vi "CopyToZip.vi"(4 "FTP Client":u16(ring) items=["VMMC", "U_HI", "Sloan Kett", "Columbia", "RRI Test"], 7 "directory path":path=path "D:/") -> ()   [LabVIEW 2022 SP3]
uses:
  <vilib>/Utility/SMTP/NI_SMTPEmail.lvlib
panel:
  out "spreadsheet string":string
  # "Save to Zip in progress. Report errors to RRI."
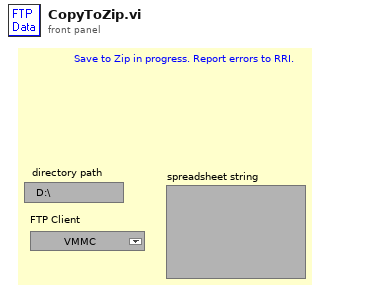
[diagram p1: front panel]
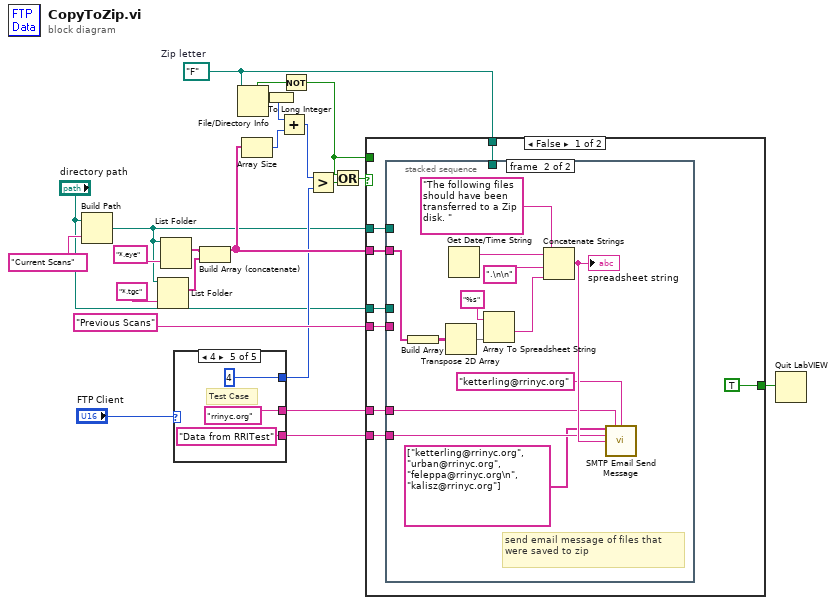
[diagram p0: block diagram]
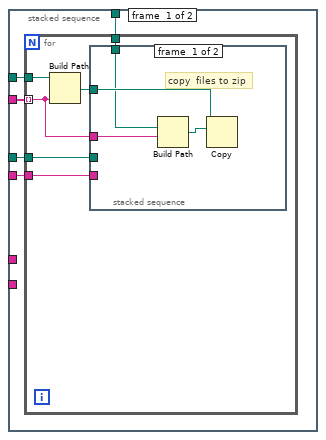
[diagram p2: hidden frame]
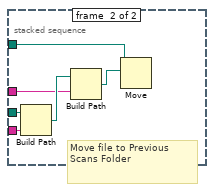
[diagram p3: hidden frame]
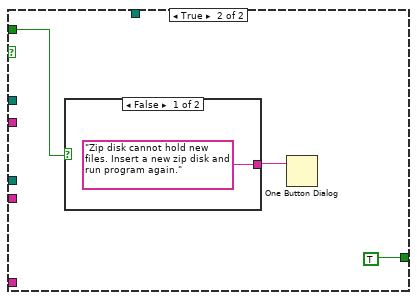
[diagram p4: hidden frame]
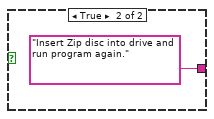
[diagram p5: hidden frame]
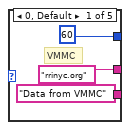
[diagram p6: hidden frame]
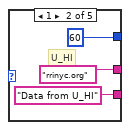
[diagram p7: hidden frame]
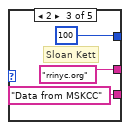
[diagram p8: hidden frame]
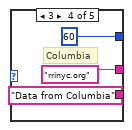
[diagram p9: hidden frame]
diagram:
  w15 = path "F:/"  # Zip letter
  n1 = Build Path(base path="directory path", name or relative path="Current Scans") -> (appended path=w9:path)
  n2 = List Folder(path=w9, pattern="*.tgc") -> (filenames=w18:string[])  [unwired: 1 in, 4 out]
  n3 = List Folder(path=w9, pattern="*.eye") -> (filenames=w19:string[])  [unwired: 1 in, 4 out]
  n4 = case shown="4" "FTP Client" {
    tunnel: ["Data from VMMC" "Data from U_HI" "Data from MSKCC" "Data from Columbia" "Data from RRITest"] -> w17
    tunnel: ["rrinyc.org" "rrinyc.org" "rrinyc.org" "rrinyc.org" "rrinyc.org"] -> w16
    tunnel: [60 60 100 60 4] -> w10
    frame 0, Default {
      # "VMMC"
    }
    frame 1 {
      # "U_HI"
    }
    frame 2 {
      # "Sloan Kett"
    }
    frame 3 {
      # "Columbia"
    }
    frame 4 {
      # "Test Case"
    }
  }
  n5 = Build Array (concatenate)(w19, w18) -> (w14:string[])
  n6 = File/Directory Info(path=w15) -> (directory=w5:bool, size=w1:i64)  [unwired: 1 in, 5 out]
  n7 = Array Size(array=w14) -> (size(s)=w12:i32)
  n8 = To Long Integer(number=w1) -> (32bit integer=w13:i32)
  n9 = Add(x=w13, y=w12) -> (x+y=w11:i32)
  n10 = Not(x=w5) -> (.not. x?=w2:bool)
  n11 = Greater?(x=w11, y=w10) -> (0:w3:bool)
  n12 = Or(x=w2, y=w3) -> (x .or. y?=w4:bool)
  n13 = case shown="False" w4 {
    tunnel: w9 -> [w46 _]
    tunnel: "Previous Scans" -> [w45 _]
    tunnel: w17 -> [w44 _]
    tunnel: w16 -> [w43 _]
    tunnel: w15 -> [w42 _]
    tunnel: w14 -> [w41 _]
    tunnel: [TRUE TRUE] -> w7
    tunnel: "directory path" -> [w39 _]
    tunnel: w2 -> [_ w81]
    frame False {
      n14 = stacked-sequence {
        tunnel: w45 -> [w51 _]
        tunnel: w46 -> [w50 _]
        tunnel: w41 -> [w49 w80]
        tunnel: w44 -> [_ w70]
        tunnel: w43 -> [_ w69]
        tunnel: w42 -> [w48 _]
        tunnel: w39 -> [w47 _]
        frame #0 {
          n15 = for {
            tunnel: w49 -> [w55] mode=indexing
            tunnel: w50 -> [w53]
            tunnel: w51 -> [w56]
            tunnel: w48 -> [w54]
            tunnel: w47 -> [w52]
            n16 = Build Path(base path=w53, name or relative path=w55) -> (appended path=w57:path)
            n17 = stacked-sequence {
              tunnel: w57 -> [w61 w62]
              tunnel: w52 -> [_ w67]
              tunnel: w56 -> [_ w66]
              tunnel: w55 -> [w60 w63]
              tunnel: w54 -> [w58 _]
              frame #0 {
                # "copy  files to zip"
                n18 = Build Path(base path=w58, name or relative path=w60) -> (appended path=w59:path)
                n19 = Copy(10:w59, 11:w61) -> ()  [unwired: 1 in, 5 out]
              }
              frame #1 {
                # "Move file to Previous Scans Folder"
                n20 = Build Path(base path=w67, name or relative path=w66) -> (appended path=w65:path)
                n21 = Build Path(base path=w65, name or relative path=w63) -> (appended path=w64:path)
                n22 = Move(source path=w62, 10:w64) -> ()  [unwired: 1 in, 5 out]
              }
            }
          }
        }
        frame #1 {
          # "send email message of files that were saved to zip"
          n23 = Build Array(w80) -> (w79:string[][])
          n24 = Transpose 2D Array(2D array=w79) -> (transposed array=w77:string[][])
          n25 = Get Date/Time String() -> (date string=w75:string)  [unwired: 4 out]
          n26 = Array To Spreadsheet String(array=w77, 3:"%s" ("format string")) -> (spreadsheet string=w73:string)  [unwired: 1 out]
          n27 = Concatenate Strings("The following files should have been transferred to a Zip disk. ", w75, ".\n\n", w73) -> (w72:string)
          "spreadsheet string" <- w72
          n28 = call <vilib>:"SMTP Email Send Message.vi"("recipients"=string[] ["ketterling@rrinyc.org", "urban@rrinyc.org", "feleppa@rrinyc.org\n", "kalisz@rrinyc.org"], "mail server"=w69, "return address"="ketterling@rrinyc.org", "subject ([No Subject])"=w70, "message"=w72) -> ()  [unwired: 1 in, 10 out]
        }
      }
    }
    frame True {
      n29 = case shown="False" w81 {
        tunnel: ["Zip disk cannot hold new files. Insert a new zip disk and run program again." "Insert Zip disc into drive and run program again."] -> w83
        frame False {
        }
        frame True {
        }
      }
      n30 = One Button Dialog(message=w83) -> ()  [unwired: 2 out]
    }
  }
  n31 = Quit LabVIEW(quit? (T)=w7) -> ()
